vi "Send_amplitude_return_voltages.vi"(5 "output cluster":T1 {"TimeStamp" format="%.2f"}, 6 "error in (no error)":errorcluster, 7 "Command":string="TIME", 8 "test response?":bool, 9 "Expected response":string) -> (0 "error IO":errorcluster, 1 "Return value":string)   [LabVIEW 2020]
uses:
  DataSocketCluster external.ctl
  vi Mode external.ctl
  04bf3837-9317-4129-9531-d6752085829f.vi
  <vilib>/Utility/error.llb/Error Cluster From Error Code.vi
  <vilib>/ErrorRing/Error Ring.xnode
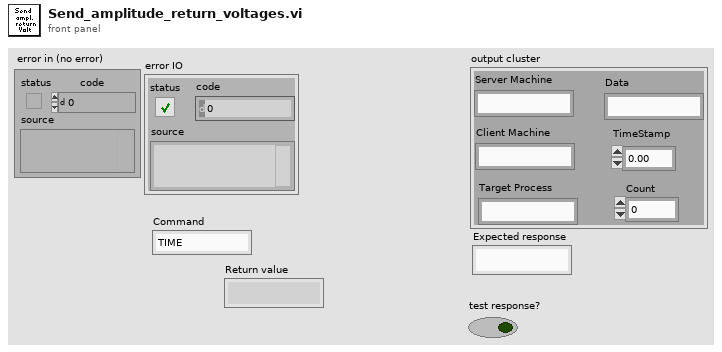
[diagram p1: front panel]
types:
  T1 = typedef "DataSocketCluster external.ctl" = cluster{"Server Machine":string, "Client Machine":string, "Data":string, "TimeStamp":dbl, "Count":i32, "Target Process":string}
  T2 = typedef "vi Mode external.ctl" = enum16{"Client", "Server"}
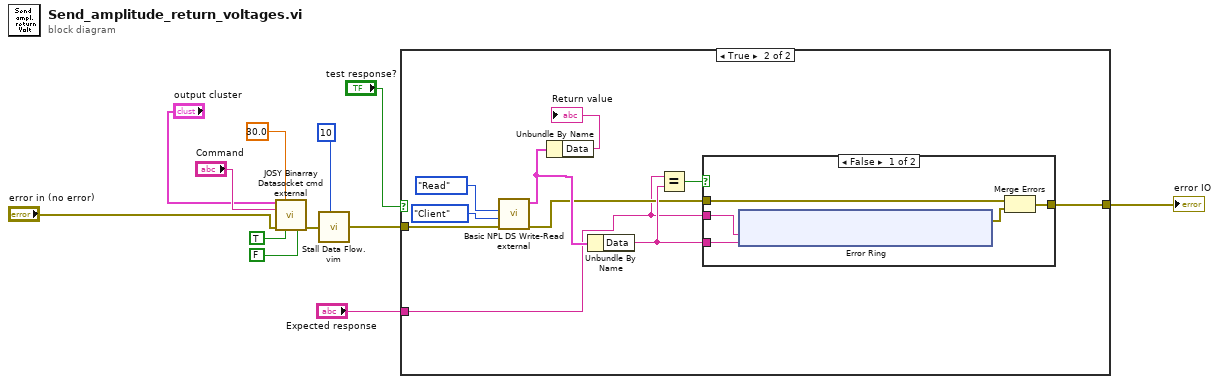
[diagram p0: block diagram]
diagram:
  n1 = call "JOSY Binarray Datasocket cmd external.vi"("DataSocketCluster In"="output cluster", "TimeOut Time (s)"=30.0, "Command"="Command", "error in (no error)"="error in (no error)", "Command has variable"=TRUE, "String"=FALSE) -> ("error out"=w9:errorcluster)  [unwired: 6 in, 3 out]
  n2 = call "Stall Data Flow.vim"("value in"=w9, "milliseconds to wait"=u32 10) -> ("value out"=w8:errorcluster)  [unwired: 1 out]
  n3 = case shown="True" "test response?" {
    tunnel: w8 -> [w13 w23]
    tunnel: [w13 w17] -> w4
    tunnel: "Expected response" -> [_ w14]
    frame False {
    }
    frame True {
      n4 = call "Basic NPL DS Write-Read external.vi"("error in (no error)"=w23, "Server Mode"=vi_Mode_external."Client", "Operation Mode"=enum16{"Read", "Write", "Write/Read"}."Read") -> ("error out"=w15:errorcluster, "DataSocketCluster Out"=w16:T1)  [unwired: 4 in, 1 out]
      n5 = Unbundle By Name(w16) -> ("Data"=→"Return value":string)
      n6 = Unbundle By Name(w16) -> ("Data"=w18:string)
      n7 = Equal?(x=w14, y=w18) -> (x = y?=w19:bool)
      n8 = case shown="False" w19 {
        tunnel: w15 -> [w25 w37]
        tunnel: w14 -> [w28 _]
        tunnel: w18 -> [w27 _]
        tunnel: [w24 w37] -> w17
        frame False {
          n9 = xnode "Error Ring"("parameter 0"=w28, "parameter 1"=w27) -> ("error out"=w26:errorcluster)
          n10 = Merge Errors(w25, w26) -> (w24:errorcluster)
        }
        frame True {
        }
      }
    }
  }
  "error IO" <- w4
